vi "DAQ Initialization.vi"(7 "queue in":refnum<queue>, 8 "error in":errorcluster, 11 "class objects in":T1) -> (0 "error out":errorcluster, 3 "Class objects":T1, 5 "queue out":refnum<queue>)   [LabVIEW 2011]
uses:
  Controls/Class Objects.ctl
  Modules/File/Configuration/Configuration.lvclass
  Modules/Hardware/Power Supply/Power Supply.lvclass
  Modules/Hardware/Mass Flow Controller/Mass Flow Controller.lvclass
  Modules/Hardware/PID/PID.lvclass
  Modules/Hardware/Valve Controller/Valve Controller.lvclass
  Modules/Hardware/Multimeter/Multimeter.lvclass
  Modules/Hardware/Vapour Generator/Vapour Generator.lvclass
  Modules/File/TDMS/TDMS.lvclass
  Controls/User Event Control.ctl
  Controls/User Event Action.ctl
  Functional Global Data/Globals.ctl
  Controls/User Interface Action.ctl
  Functional Global Data/Run Data.ctl
  Modules/Menu/Menu Action.ctl
  Controls/Class Labels.ctl
  Controls/TDMS File Handling.ctl
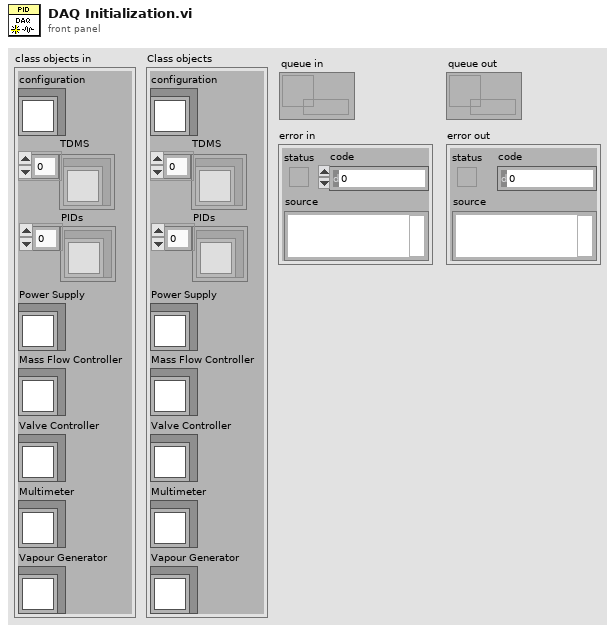
[diagram p1: front panel]
types:
  T1 = typedef "Class Objects.ctl" = cluster{"configuration":refnum<class "Configuration.lvclass">, "TDMS":refnum<class "TDMS.lvclass">[], "Power Supply":refnum<class "Power Supply.lvclass">, "Mass Flow Controller":refnum<class "Mass Flow Controller.lvclass">, "Valve Controller":refnum<class "Valve Controller.lvclass">, "Multimeter":refnum<class "Multimeter.lvclass">, "Vapour Generator":refnum<class "Vapour Generator.lvclass">, "PIDs":refnum<class "PID.lvclass">[]}
  T2 = typedef "Globals.ctl" = enum16{"Initialize", "Get DAQ Params", "Get Data Display Params", "Set DAQ Params", "Set Data Display Params"}
  T3 = typedef "User Interface Action.ctl" = enum16{"Initialize", "Data Acquisition Disable", "Data View Disable", "Sample Set", "Sample Set 2D Data", "Sample Set x0 & dx", "Sample Add", "Sample Set Cursor", "Sample Set Offset & Multiplier", "Sample Set Axis Labels", "Sample Parameters Disabled", "Sample Parameters Update", "Run Update", "Run Set Offset & Multiplier", "Run Set Axis Labels", "Run Set Cursor", "Run Set Disabled", "Run Parameters Update", "Run Parameters Disabled", "Run Number Set", "Run Number Set Range", "Run Number Set Disabled", "Sample Number Set", "Sample Number Set Range", "Notes Set Value", "Update Plot", "Set Plot Parameters", "Update Concentration Plot", "Time Set", "Clear DAQ Display", "Clear Analysis Display", "Status Bar Set", "Progress Bar Set", "Display Mode Set", "Experiment Type Set", "Analysis Plot Average Set", "Stop"}
  T4 = enum8{"Enabled", "Disabled", "Disabled and Grayed Out"}
  T5 = typedef "Run Data.ctl" = enum16{"Initialize", "Add Sample Channel", "Set Run", "Get Number of Runs", "Set Run Params", "Get Spectrum", "Get Run Params", "Get Sample Params", "Get History", "Get Averaged History", "Get Run Param Names", "Set Run Param Names", "Get Sample Param Names", "Set Sample Param Names", "Get MFC Flow Rate Challenge Profile", "Get History Average"}
  T6 = typedef "Menu Action.ctl" = enum16{"Initialize", "Insert Item", "Remove Item", "Set Checked Item", "Get Checked Item", "Get Item Index", "Item Present?", "Stop"}
  T7 = typedef "User Event Control.ctl" = cluster{"action":T8, "data":variant}
  T8 = typedef "User Event Action.ctl" = enum16{"Program Initialization", "Device Connections", "Device Settings", "Options", "DAQ Init", "PID Sample Test", "PID with PS Challenge", "PID with MFC Challenge", "Multimeter Sample Test", "Multimeter with MFC Challenge", "DAQ Stop", "Open Data File", "View Data File", "Change Display Mode", "Load INL PID Run Data", "Load Baseline-Mocon PID Data", "Load Multimeter Data", "Set Channel Sample", "Key Down", "Add Spectrum to Plot", "Add History to Plot", "Export History to Excel", "Clear Plots", "Save Plot", "Save Spectral Variable", "History Cursor Release", "Analysis Plot Cursor Release", "Program Deinitialization"}
  T9 = typedef "Class Labels.ctl" = enum16{"Configuration", "TDMS", "PID", "Power Supply", "Vapour Generator", "MFC", "NMR", "Valve Controller", "Multimeter"}
  T10 = typedef "TDMS File Handling.ctl" = enum16{"Add TDMS File", "Get Active TDMS File", "Set Active TDMS File", "Set Active TDMS File Index"}
  T11 = typedef "Data Acquisition Parameters.ctl" = cluster{"Experiment Type":T12, "Experiment Name":string, "Operator Name":string, "Notes":string, "TDMS File Path":path, "Data Acquisition State":bool, "PID Voltage Sweep":T13, "MFC Challenge Profile - Heaviside Step":T14, "MFC Challenge Profile":T15, "MFC Challenge Profile - Staircase":T16}
  T12 = typedef "DAQ Type.ctl" = enum16{"PID Sample", "PID with PS Challenge", "PID with MFC Challenge", "Multimeter Sample", "Multimeter with MFC Challenge"}
  T13 = typedef "PID Voltage Seep Settings.ctl" = cluster{"Voltage Step (V)":dbl, "Voltage Range (V)":cluster{u16, u16}, "Time Step (s)":dbl, "Voltage Step Direction":enum16{"High 2 Low", "Low 2 High"}}
  T14 = typedef "MFC Challenge Profile - Heaviside Step.ctl" = cluster{"Valve Open Duration":u16, "MFC Flow Rate":dbl, "Valve Open Repeats":u16, "Valve Open Start":u16}
  T15 = typedef "MFC Challen Profile Type.ctl" = enum16{"Heaviside", "Staircase"}
  T16 = typedef "MFC Challenge Profile - Staircase.ctl" = cluster{"Step Time Duration":u16, "Step Flow Rate":dbl, "Steps":u16, "Valve Open Start":u16, "Recovery":bool, "Repeats":u16}
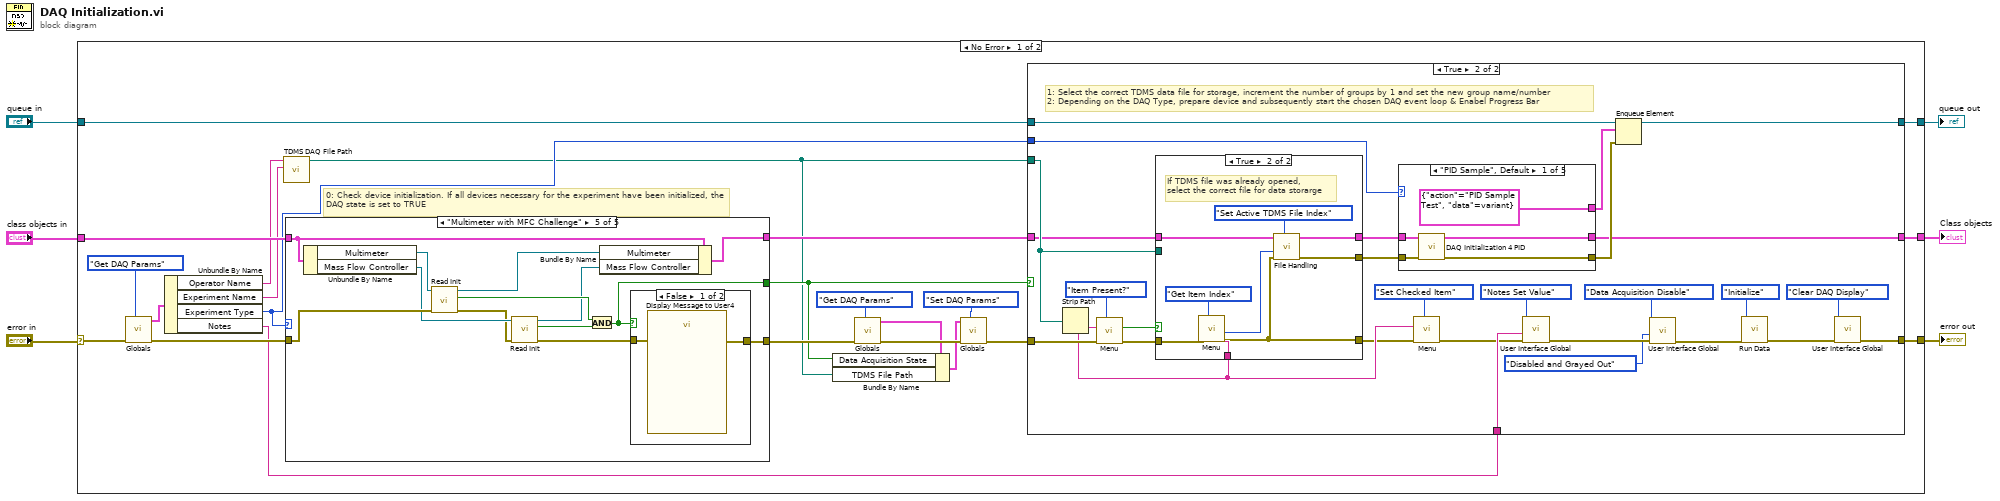
[diagram p0: block diagram]
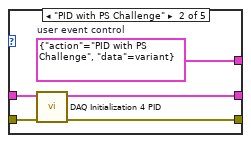
[diagram p3: hidden frame]
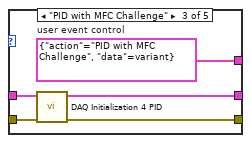
[diagram p4: hidden frame]
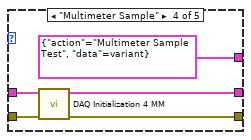
[diagram p5: hidden frame]
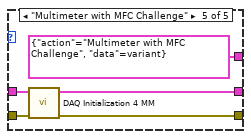
[diagram p6: hidden frame]
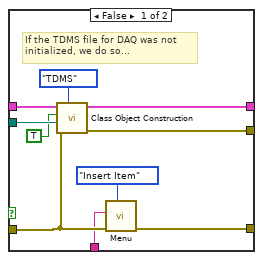
[diagram p7: hidden frame]
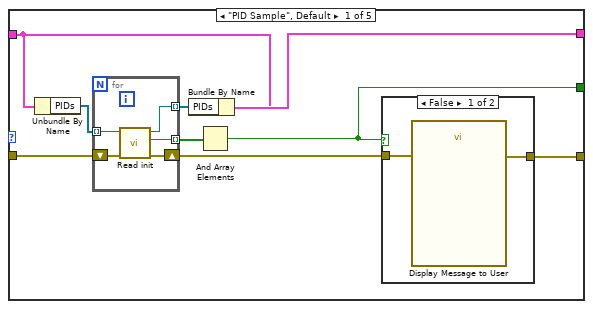
[diagram p8: hidden frame]
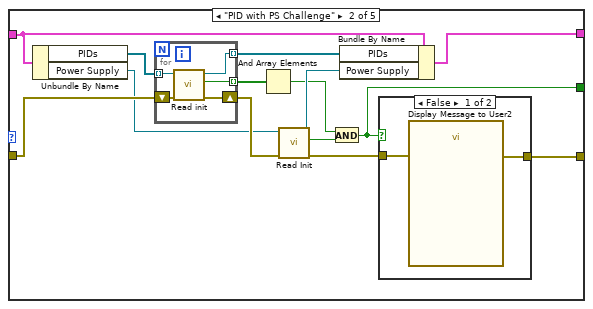
[diagram p10: hidden frame]
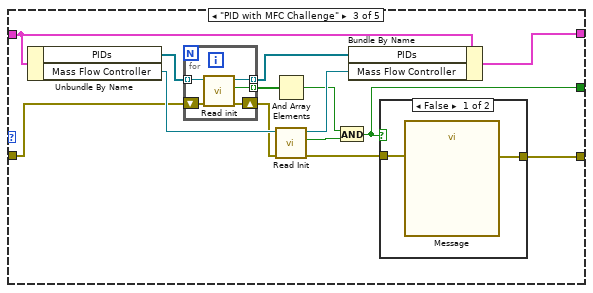
[diagram p12: hidden frame]
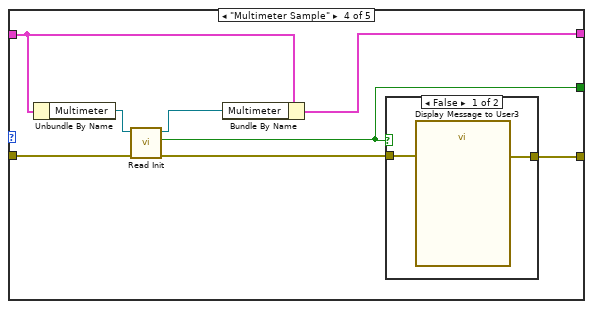
[diagram p14: hidden frame]
diagram:
  n1 = case shown="No Error" "error in" {
    selector: "error in" -> [w13 w193]
    tunnel: [w29 w193] -> w6
    tunnel: [w28 w194] -> w5
    tunnel: "class objects in" -> [w24 w194]
    tunnel: [w14 w195] -> w3
    tunnel: "queue in" -> [w12 w195]
    frame No Error {
      # "0: Check device initialization. If all devices necessary for the experiment have been initialized, the DAQ state is set to TRUE"
      n2 = call "Globals.vi"("action"=Globals."Get DAQ Params", "error in"=w13) -> ("error out"=w25:errorcluster, "Data Acquisition"=w27:T11)  [unwired: 7 in, 1 out]
      n3 = Unbundle By Name(w27) -> ("Operator Name"=w11:string, "Experiment Name"=w10:string, "Experiment Type"=w23:T12, "Notes"=w7:string)
      n4 = call "TDMS DAQ File Path.vi"("Experiment Name"=w10, "Operator Name"=w11) -> ("appended path"=w9:path)  [unwired: 9 in]
      n5 = case shown="\"Multimeter with MFC Challenge\"" w23 {
        tunnel: [w111 w130 w152 w169 w178] -> w15
        tunnel: [w113 w132 w156 w171 w180] -> w18
        tunnel: [w105 w131 w153 w170 w177] -> w17
        tunnel: w24 -> [w110 w129 w149 w168 w181]
        tunnel: w25 -> [w109 w128 w150 w167 w187]
        frame "PID Sample", Default {
          n6 = Unbundle By Name(w110) -> ("PIDs"=w108:refnum<class "PID.lvclass">[])
          n7 = for {
            tunnel: [w118] -> w106 mode=indexing
            tunnel: w108 -> [w116] mode=indexing
            tunnel: [w115] -> w107 mode=indexing
            shift-right: [w114] -> w112
            shift-left: w109 -> [w117]
            n8 = call-dynamic "Read init.vi"("error in (no error)"=w117, "Detector in"=w116) -> ("error out"=w114:errorcluster, "init"=w118:bool, "Detector out"=w115:refnum<class "PID.lvclass">)  [unwired: 7 in]
          }
          n9 = Bundle By Name(cluster=w110, "PIDs"=w107) -> (w111:T1)
          n10 = And Array Elements(Boolean array=w106) -> (logical AND=w105:bool)
          n11 = case shown="False" w105 {
            tunnel: w112 -> [w120 w121]
            tunnel: [w119 w121] -> w113
            frame False {
              n12 = call "Display Message to User"("error in (no error)"=w120) -> ("error out"=w119:errorcluster)  [unwired: 9 in, 1 out]
            }
            frame True {
            }
          }
        }
        frame "PID with PS Challenge" {
          n13 = Unbundle By Name(w129) -> ("PIDs"=w127:refnum<class "PID.lvclass">[], "Power Supply"=w123:refnum<class "Power Supply.lvclass">)
          n14 = for {
            tunnel: [w140] -> w126 mode=indexing
            tunnel: w127 -> [w138] mode=indexing
            shift-right: [w137] -> w124
            shift-left: w128 -> [w139]
            tunnel: [w136] -> w122 mode=indexing
            n15 = call-dynamic "Read init.vi"("error in (no error)"=w139, "Detector in"=w138) -> ("error out"=w137:errorcluster, "init"=w140:bool, "Detector out"=w136:refnum<class "PID.lvclass">)  [unwired: 7 in]
          }
          n16 = And Array Elements(Boolean array=w126) -> (logical AND=w125:bool)
          n17 = call-dynamic "Read Init.vi"("error in (no error)"=w124, "Power Supply in"=w123) -> ("error out"=w133:errorcluster, "Init"=w134:bool, "Power Supply out"=w135:refnum<class "Power Supply.lvclass">)  [unwired: 7 in]
          n18 = And(x=w125, y=w134) -> (x .and. y?=w131:bool)
          n19 = Bundle By Name(cluster=w129, "PIDs"=w122, "Power Supply"=w135) -> (w130:T1)
          n20 = case shown="False" w131 {
            tunnel: w133 -> [w142 w143]
            tunnel: [w141 w143] -> w132
            frame False {
              n21 = call "Display Message to User2"("error in (no error)"=w142) -> ("error out"=w141:errorcluster)  [unwired: 9 in, 1 out]
            }
            frame True {
            }
          }
        }
        frame "PID with MFC Challenge" {
          n22 = Unbundle By Name(w149) -> ("PIDs"=w148:refnum<class "PID.lvclass">[], "Mass Flow Controller"=w151:refnum<class "Mass Flow Controller.lvclass">)
          n23 = for {
            tunnel: [w162] -> w145 mode=indexing
            tunnel: w148 -> [w160] mode=indexing
            shift-right: [w158] -> w146
            shift-left: w150 -> [w161]
            tunnel: [w159] -> w147 mode=indexing
            n24 = call-dynamic "Read init.vi"("error in (no error)"=w161, "Detector in"=w160) -> ("error out"=w158:errorcluster, "init"=w162:bool, "Detector out"=w159:refnum<class "PID.lvclass">)  [unwired: 7 in]
          }
          n25 = And Array Elements(Boolean array=w145) -> (logical AND=w144:bool)
          n26 = call-dynamic "Read Init.vi"("error in (no error)"=w146, "Mass Flow Controller in"=w151) -> ("error out"=w155:errorcluster, "Init"=w154:bool, "Mass Flow Controller out"=w157:refnum<class "Mass Flow Controller.lvclass">)  [unwired: 7 in]
          n27 = And(x=w144, y=w154) -> (x .and. y?=w153:bool)
          n28 = Bundle By Name(cluster=w149, "PIDs"=w147, "Mass Flow Controller"=w157) -> (w152:T1)
          n29 = case shown="False" w153 {
            tunnel: w155 -> [w164 w165]
            tunnel: [w163 w165] -> w156
            frame False {
              n30 = call "Message"("error in (no error)"=w164) -> ("error out"=w163:errorcluster)  [unwired: 9 in, 1 out]
            }
            frame True {
            }
          }
        }
        frame "Multimeter Sample" {
          n31 = Unbundle By Name(w168) -> ("Multimeter"=w166:refnum<class "Multimeter.lvclass">)
          n32 = call-dynamic "Read Init.vi"("error in (no error)"=w167, "Multimeter in"=w166) -> ("error out"=w172:errorcluster, "Init"=w170:bool, "Multimeter out"=w173:refnum<class "Multimeter.lvclass">)  [unwired: 7 in]
          n33 = Bundle By Name(cluster=w168, "Multimeter"=w173) -> (w169:T1)
          n34 = case shown="False" w170 {
            tunnel: w172 -> [w175 w176]
            tunnel: [w174 w176] -> w171
            frame False {
              n35 = call "Display Message to User3"("error in (no error)"=w175) -> ("error out"=w174:errorcluster)  [unwired: 9 in, 1 out]
            }
            frame True {
            }
          }
        }
        frame "Multimeter with MFC Challenge" {
          n36 = Unbundle By Name(w181) -> ("Multimeter"=w188:refnum<class "Multimeter.lvclass">, "Mass Flow Controller"=w186:refnum<class "Mass Flow Controller.lvclass">)
          n37 = call-dynamic "Read Init.vi"("error in (no error)"=w187, "Multimeter in"=w188) -> ("error out"=w185:errorcluster, "Init"=w184:bool, "Multimeter out"=w189:refnum<class "Multimeter.lvclass">)  [unwired: 7 in]
          n38 = call-dynamic "Read Init.vi"("error in (no error)"=w185, "Mass Flow Controller in"=w186) -> ("error out"=w179:errorcluster, "Init"=w183:bool, "Mass Flow Controller out"=w182:refnum<class "Mass Flow Controller.lvclass">)  [unwired: 7 in]
          n39 = And(x=w184, y=w183) -> (x .and. y?=w177:bool)
          n40 = Bundle By Name(cluster=w181, "Multimeter"=w189, "Mass Flow Controller"=w182) -> (w178:T1)
          n41 = case shown="False" w177 {
            tunnel: w179 -> [w191 w192]
            tunnel: [w190 w192] -> w180
            frame False {
              n42 = call "Display Message to User4"("error in (no error)"=w191) -> ("error out"=w190:errorcluster)  [unwired: 9 in, 1 out]
            }
            frame True {
            }
          }
        }
      }
      n43 = call "Globals.vi"("action"=Globals."Get DAQ Params", "error in"=w18) -> ("error out"=w22:errorcluster, "Data Acquisition"=w8:T11)  [unwired: 7 in, 1 out]
      n44 = Bundle By Name(cluster=w8, "Data Acquisition State"=w17, "TDMS File Path"=w9) -> (w21:T11)
      n45 = call "Globals.vi"("action"=Globals."Set DAQ Params", "error in"=w22, "Data Acquisition"=w21) -> ("error out"=w16:errorcluster)  [unwired: 6 in, 2 out]
      n46 = case shown="True" w17 {
        tunnel: [w30 w33] -> w29
        tunnel: [w31 w36] -> w28
        tunnel: w9 -> [_ w60]
        tunnel: w23 -> [_ w49]
        tunnel: w16 -> [w30 w59]
        tunnel: w15 -> [w31 w58]
        tunnel: w12 -> [w32 w48]
        tunnel: [w32 w37] -> w14
        tunnel: w7 -> [_ w43]
        frame False {
        }
        frame True {
          # "1: Select the correct TDMS data file for storage, increment the number of groups by 1 and set the new group name/number\n2: Depending on the DAQ Type, prepare device and subsequently start the chosen DAQ event loop & Enabel Progress Bar"
          n47 = Strip Path(path=w60) -> (name=w57:string)  [unwired: 1 out]
          n48 = call "Menu.vi"("action"=Menu_Action."Item Present?" ("Menu"), "error in"=w59, "item tag"=w57) -> ("error out"=w54:errorcluster, "Item Present?"=w53:bool)  [unwired: 5 in, 2 out]
          n49 = case shown="True" w53 {
            tunnel: w54 -> [w89 w102]
            tunnel: [w88 w99] -> w55
            tunnel: w57 -> [w87 w101]
            tunnel: w60 -> [w91 _]
            tunnel: [w93 w97] -> w50
            tunnel: w58 -> [w94 w100]
            tunnel: [w92 w96] -> w51
            frame False {
              # "If the TDMS file for DAQ was not\ninitialized, we do so..."
              n50 = call "Class Object Construction.vi"("class"=Class_Labels."TDMS" ("Class"), "error in"=w89, "param2"=w91, "param 1"=TRUE, "classes in"=w94) -> ("error out"=w92:errorcluster, "classes out"=w93:T1)  [unwired: 4 in]
              n51 = call "Menu.vi"("action"=Menu_Action."Insert Item", "error in"=w89, "item tag"=w87) -> ("error out"=w88:errorcluster)  [unwired: 5 in, 3 out]
            }
            frame True {
              # "If TDMS file was already opened,\nselect the correct file for data storarge"
              n52 = call "Menu.vi"("action"=Menu_Action."Get Item Index", "error in"=w102, "item tag"=w101) -> ("error out"=w99:errorcluster, "item index"=w98:i32)  [unwired: 5 in, 2 out]
              n53 = call "File Handling.vi"("TDMS File Handling"=TDMS_File_Handling."Set Active TDMS File Index", "error in"=w99, "Active File Index"=w98, "Class objects"=w100) -> ("error out"=w96:errorcluster, "Class objects"=w97:T1)  [unwired: 5 in, 1 out]
            }
          }
          n54 = case shown="\"PID Sample\", Default" w49 {
            tunnel: [T7 {"action"=enum."PID Sample Test", "data"=variant} ("user event control") w70 w75 T7 {"action"=enum."Multimeter Sample Test", "data"=variant} ("user event control") T7 {"action"=enum."Multimeter with MFC Challenge", "data"=variant} ("user event control")] -> w47
            tunnel: w51 -> [w63 w68 w74 w79 w84]
            tunnel: w50 -> [w64 w69 w73 w78 w85]
            tunnel: [w62 w67 w72 w77 w83] -> w36
            tunnel: [w61 w66 w71 w76 w82] -> w46
            frame "PID Sample", Default {
              n55 = call "DAQ Initialization 4 PID.vi"("error in"=w63, "classes in"=w64) -> ("error out"=w61:errorcluster, "classes out"=w62:T1)  [unwired: 8 in]
            }
            frame "PID with PS Challenge" {
              w70 = T7 {"action"=enum."PID with PS Challenge", "data"=variant}  # user event control
              n56 = call "DAQ Initialization 4 PID.vi"("error in"=w68, "classes in"=w69) -> ("error out"=w66:errorcluster, "classes out"=w67:T1)  [unwired: 8 in]
            }
            frame "PID with MFC Challenge" {
              w75 = T7 {"action"=enum."PID with MFC Challenge", "data"=variant}  # user event control
              n57 = call "DAQ Initialization 4 PID.vi"("error in"=w74, "classes in"=w73) -> ("error out"=w71:errorcluster, "classes out"=w72:T1)  [unwired: 8 in]
            }
            frame "Multimeter Sample" {
              n58 = call "DAQ Initialization 4 MM.vi"("error in"=w79, "classes in"=w78) -> ("error out"=w76:errorcluster, "classes out"=w77:T1)  [unwired: 8 in]
            }
            frame "Multimeter with MFC Challenge" {
              n59 = call "DAQ Initialization 4 MM.vi"("error in"=w84, "classes in"=w85) -> ("error out"=w82:errorcluster, "classes out"=w83:T1)  [unwired: 8 in]
            }
          }
          n60 = call "Menu.vi"("action"=Menu_Action."Set Checked Item" ("Menu"), "error in"=w55, "item tag"=w57) -> ("error out"=w42:errorcluster)  [unwired: 5 in, 3 out]
          n61 = call "User Interface Global.vi"("error in"=w42, "data1"=w43, "action"=User_Interface_Action."Notes Set Value") -> ("error out"=w40:errorcluster)  [unwired: 8 in]
          n62 = Enqueue Element(queue=w48, element=w47, error in (no error)=w46) -> (queue out=w37:refnum<queue>)  [unwired: 1 in, 2 out]
          n63 = call "User Interface Global.vi"("error in"=w40, "data1"=T4."Disabled and Grayed Out" ("Disabled"), "action"=User_Interface_Action."Data Acquisition Disable") -> ("error out"=w38:errorcluster)  [unwired: 8 in]
          n64 = call "Run Data.vi"("error in"=w38, "action"=Run_Data."Initialize" ("Action")) -> ("error out"=w34:errorcluster)  [unwired: 6 in, 3 out]
          n65 = call "User Interface Global.vi"("error in"=w34, "action"=User_Interface_Action."Clear DAQ Display") -> ("error out"=w33:errorcluster)  [unwired: 9 in]
        }
      }
    }
    frame Error {
    }
  }
  "error out" <- w6
  "Class objects" <- w5
  "queue out" <- w3
